vi "Set Voltage.vi"(8 "error in (no error)":errorcluster, 10 "Voltage":dbl, 11 "4322 in":refnum<class "4322.lvclass">) -> (0 "error out":errorcluster, 3 "4322 out":refnum<class "4322.lvclass">)   [LabVIEW 2019, in "4322.lvlib" / "4322.lvclass"]
uses:
  Library/4322.lvclass
  builds/Instruments/Analog-Output.lvlibp/Library/Analog-Output.lvclass
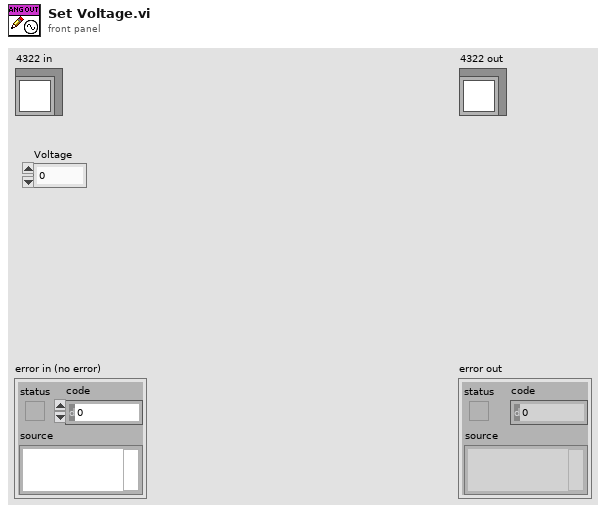
[diagram p1: front panel]
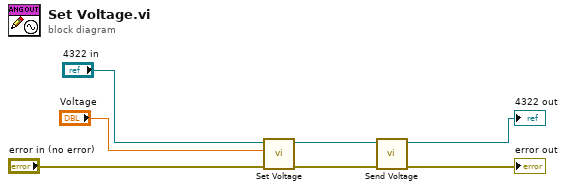
[diagram p0: block diagram]
diagram:
  n1 = call-parent "Set Voltage.vi"("error in (no error)"="error in (no error)", "Voltage"="Voltage", "Analog-Output in"="4322 in") -> ("error out"=w3:errorcluster, "Analog-Output out"=w4:refnum<class "4322.lvclass">)  [unwired: 7 in]
  n2 = call "Send Voltage.vi"("error in"=w3, "4322 in"=w4) -> ("error out"=→"error out":errorcluster, "4322 out"=→"4322 out":refnum<class "4322.lvclass">)  [unwired: 8 in]
